vi "log_ratio_test.vi"() -> ()   [LabVIEW 2013]
panel:
  out "size(s)":i32[](array[numeric])
  out "Array":sgl[][](array[numeric])
  in  "Y":i32=7
  in  "X":i32=9
  in  "Reactor":i32
  in  "DIVA DIRECTORY":path=path "D:/BDDatabase/BDData"
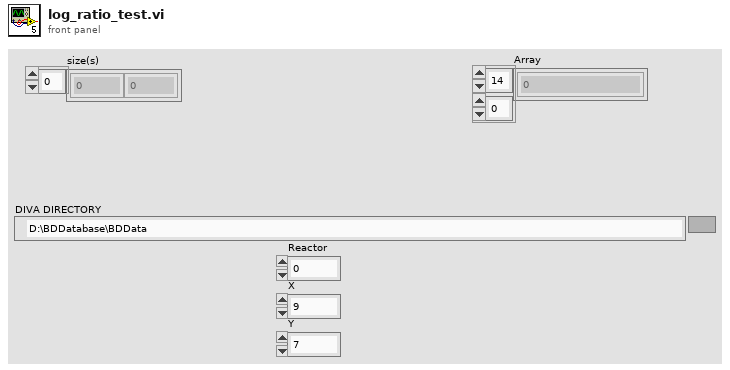
[diagram p1: front panel]
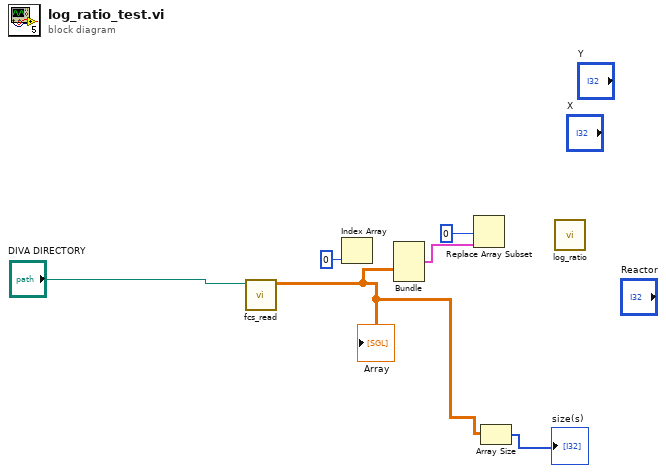
[diagram p0: block diagram]
diagram:
  n1 = call "fcs_read.vi"("Path"="DIVA DIRECTORY") -> ("Array"=w2:sgl[][])  [unwired: 7 in, 3 out]
  "Array" <- w2
  n2 = Index Array(index=0) -> ()  [unwired: 1 in, 1 out]
  n3 = Bundle("Array"=w2) -> (w5:cluster{void, void, void, "Array":sgl[][], void})  [unwired: 5 in]
  n4 = Replace Array Subset(new element=w5, index=0) -> ()  [unwired: 1 in, 1 out]
  n5 = Array Size(array=w2) -> (size(s)=→"size(s)":i32[])
  n6 = call "log_ratio.vi"() -> ()  [unwired: 10 in, 2 out]
